vi "Autonomous Independent.vi"() -> ()   [LabVIEW 2014]
doc: "This VI is called when autonomous begins, and will automatically be terminated when autonomous ends. You can carry out timed or sensor driven robot movement independently without needing to return to the caller."
uses:
  <vilib>/addons/control/pid/pid.llb/PID Output Rate Limiter (DBL).vi
  <vilib>/addons/control/pid/NI_PID_pid.lvlib
panel:
  in  "Y 8":dbl
  in  "X 8":dbl format="%#_13g"
  in  "Forward_Drive_Time 2":dbl=2.55
  in  "Y 7":dbl=0.8
  in  "X 7":dbl format="%#_13g"
  in  "Max_Speed 2":dbl=1000.0 format="%#_13g"
  in  "Y 6":dbl
  in  "X 6":dbl format="%#_13g"
  in  "Container? y_t n_f":bool=TRUE
  in  "X 5":dbl format="%#_13g"
  in  "Y 5":dbl
  in  "Numeric":dbl=1781.0 format="%#_13g"
  in  "Max_Speed":dbl=1000.0 format="%#_13g"
  in  "Y 4":dbl
  in  "X 4":dbl format="%#_13g"
  in  "Forward_Drive_Time":dbl=2.8
  in  "Y 3":dbl=0.8
  in  "X 3":dbl format="%#_13g"
  in  "Stop":dbl=0.01
  in  "output rate (EGU/min)":dbl=25.0 format="%.2f"
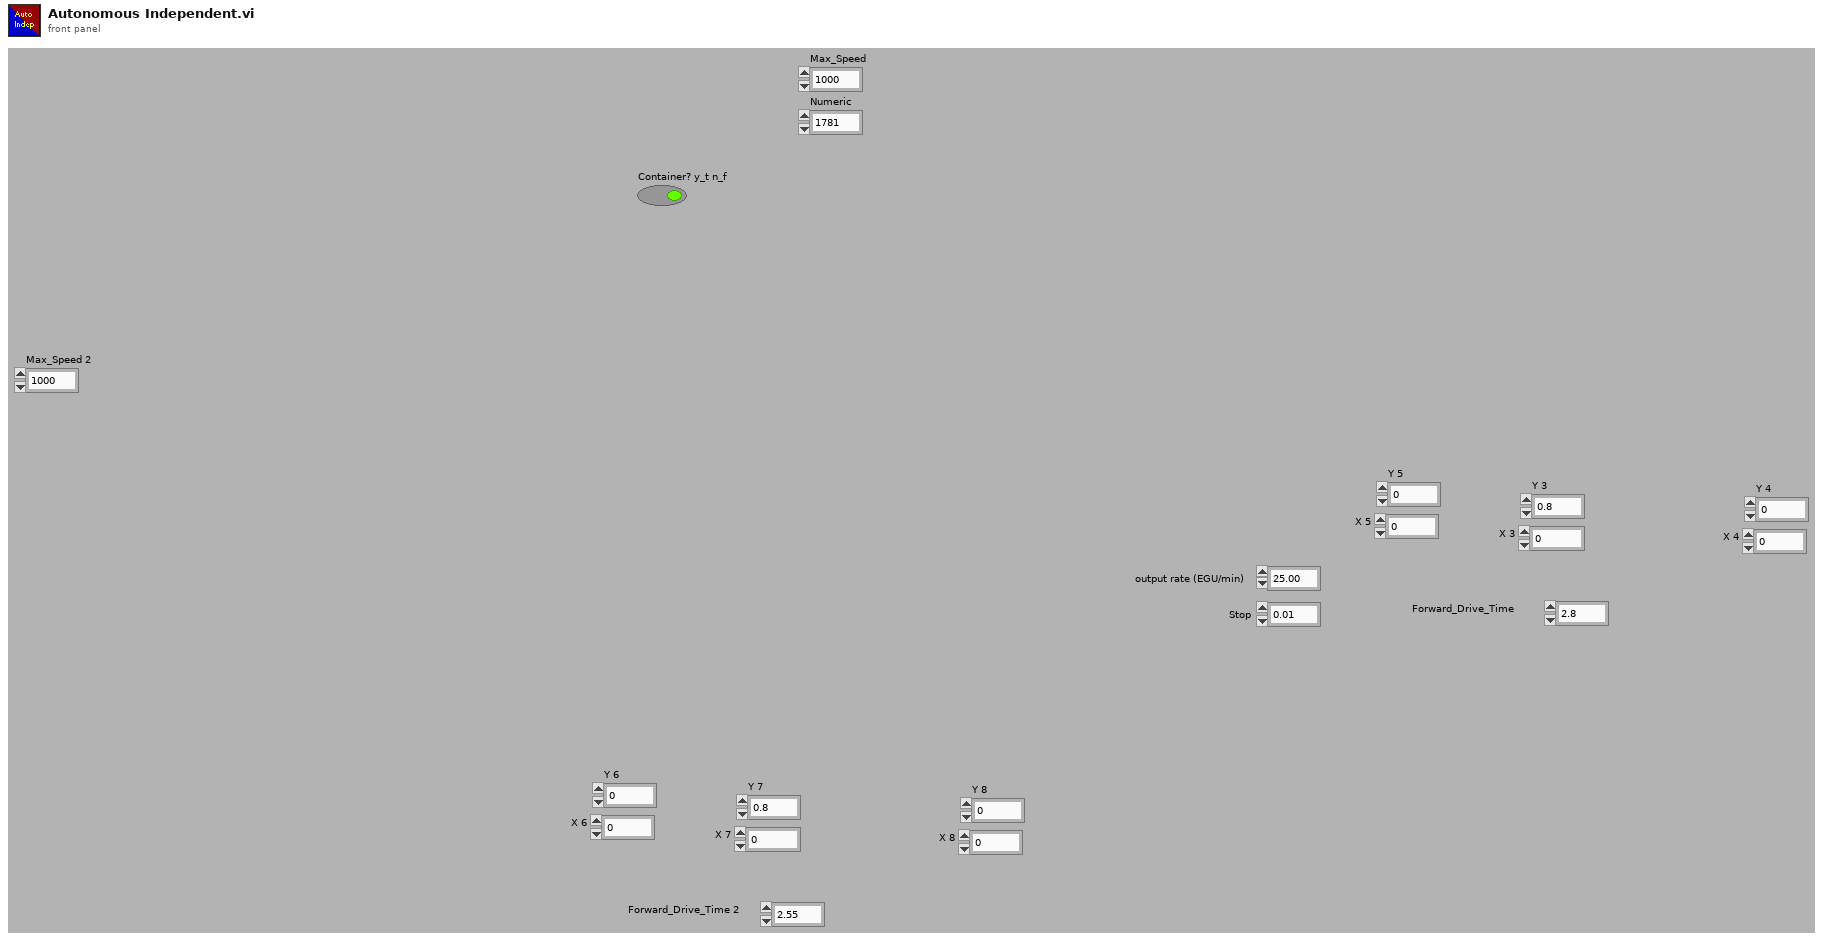
[diagram p1: front panel]
types:
  T1 = typedef "WPI_EncoderDevRef.ctl" = cluster{"DevStatus":errorcluster, "EncoderIndex":T2, "CounterIndex":T3, "DistancePerCount":dbl, "Decoding Type":T4}
  T2 = typedef "FPGA_EncoderIdx.ctl" = enum8{"Enc 0", "Enc 1", "Enc 2", "Enc 3", "Enc 4", "Enc 5", "Enc 6", "Enc 7", "Invalid"}
  T3 = typedef "FPGA_CounterCtrSystemIndex.ctl" = enum8{"Ctr 0", "Ctr 1", "Ctr 2", "Ctr 3", "Ctr 4", "Ctr 5", "Ctr 6", "Ctr 7", "Invalid"}
  T4 = typedef "WPI_EncoderType.ctl" = enum16{"1x", "2x", "4x"}
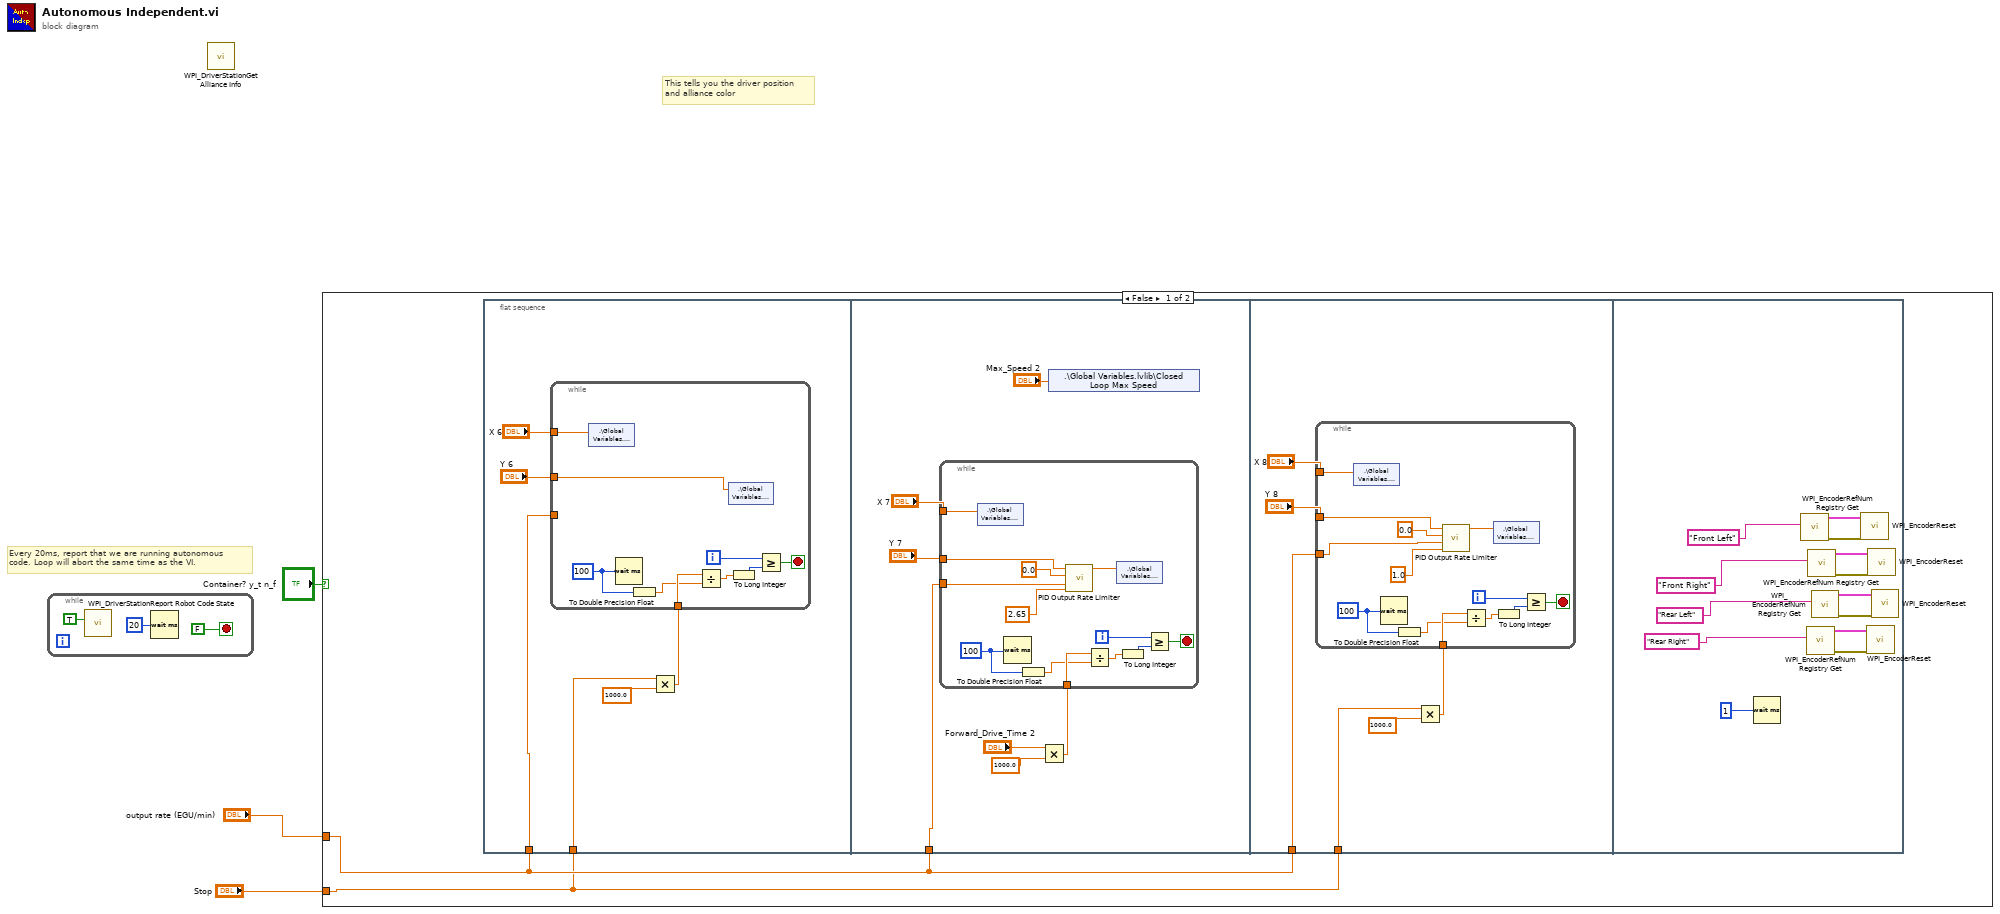
[diagram p0: block diagram]
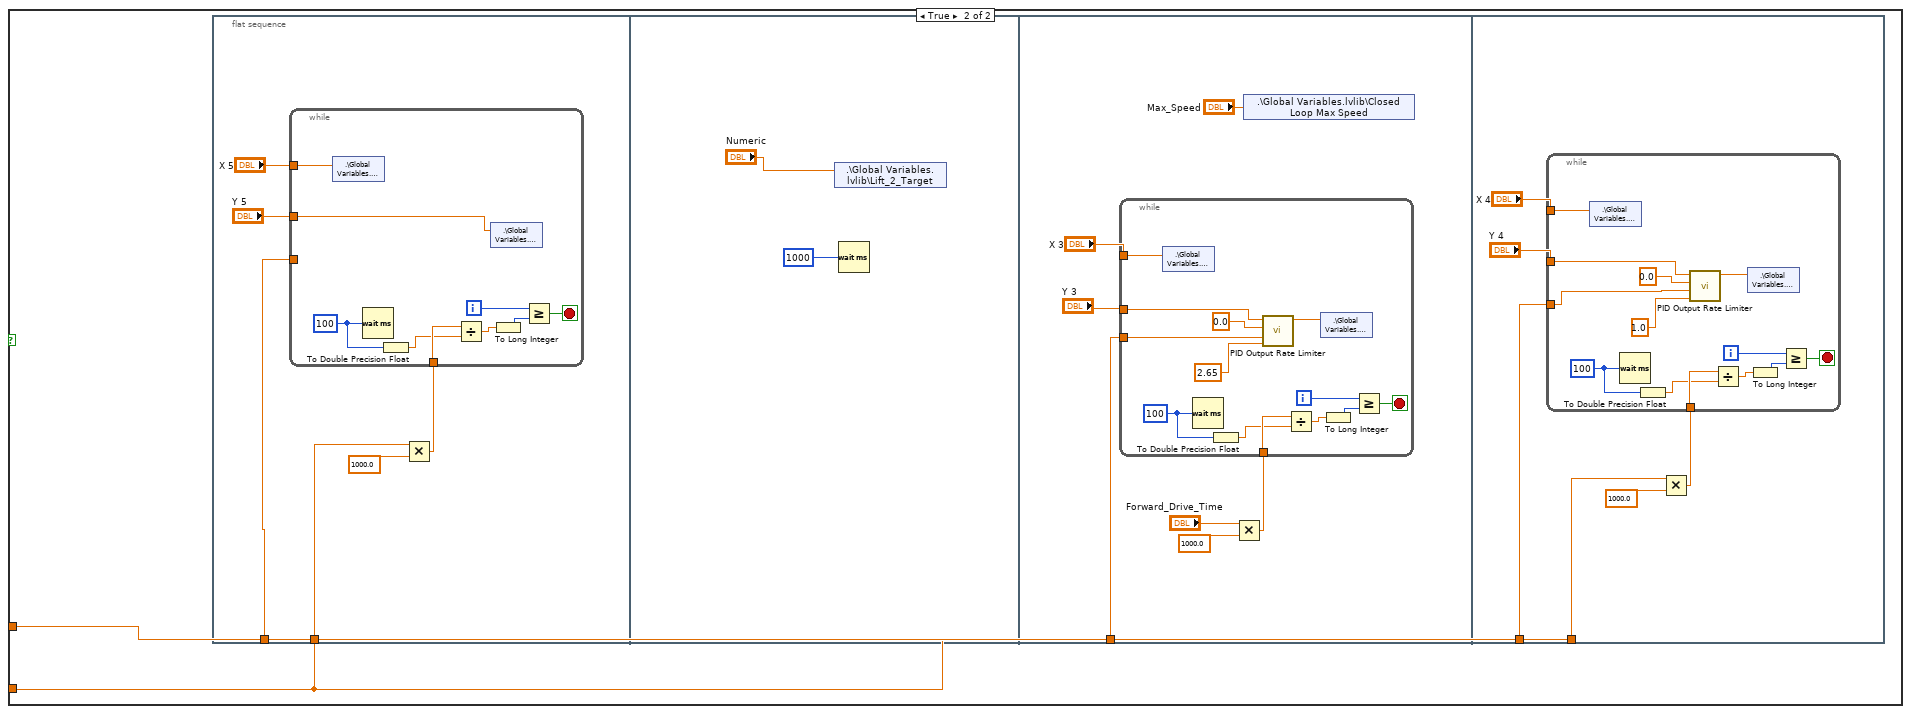
[diagram p2: hidden frame]
diagram:
  # "Every 20ms, report that we are running autonomous\ncode. Loop will abort the same time as the VI."
  # "This tells you the driver position\nand alliance color"
  n1 = while {
    stop <- FALSE stop-if-true
    n2 = call <vilib>:"WPI_DriverStationReport Robot Code State.vi"("Autonomous"=TRUE) -> ()  [unwired: 10 in, 1 out]
    n3 = Wait (ms)(milliseconds to wait=u32 20) -> ()  [unwired: 1 out]
  }
  n4 = call <vilib>:"WPI_DriverStationGet Alliance Info.vi"() -> ()  [unwired: 12 out]
  n5 = case shown="False" "Container? y_t n_f" {
    tunnel: "output rate (EGU/min)" -> [w8 w77]
    tunnel: "Stop" -> [w7 w76]
    frame False {
      n6 = flat-sequence {
        tunnel: w8 -> [w10]
        tunnel: w7 -> [w9]
        tunnel: w8 -> [w24]
        tunnel: w8 -> [w45]
        tunnel: w7 -> [w44]
        frame #0 {
          n7 = Multiply(x=w9, y=1000.0) -> (x*y=w13:dbl)
          n8 = while {
            tunnel: w13 -> [w21]
            tunnel: "X 6" -> [w16]
            tunnel: "Y 6" -> [w15]
            tunnel: w10 -> [_]
            i -> [w19]
            stop <- w23 stop-if-true
            w22 = u32 100 ("milliseconds to wait")
            n9 = shared-variable ".\\Global Variables.lvlib\\X"(w16) -> ()  [unwired: 1 in, 1 out]
            n10 = Wait (ms)(milliseconds to wait=w22) -> ()  [unwired: 1 out]
            n11 = To Double Precision Float(number=w22) -> (double precision float=w20:dbl)
            n12 = Divide(x=w21, y=w20) -> (x/y=w18:dbl)
            n13 = shared-variable ".\\Global Variables.lvlib\\Y"(w15) -> ()  [unwired: 1 in, 1 out]
            n14 = To Long Integer(number=w18) -> (32bit integer=w17:i32)
            n15 = Greater Or Equal?(x=w19, y=w17) -> (x >= y?=w23:bool)
          }
        }
        frame #1 {
          n16 = Multiply(x="Forward_Drive_Time 2", y=1000.0) -> (x*y=w27:dbl)
          n17 = while {
            tunnel: "Y 7" -> [w33]
            tunnel: w24 -> [w42]
            tunnel: w27 -> [w38]
            tunnel: "X 7" -> [w31]
            i -> [w36]
            stop <- w41 stop-if-true
            w39 = u32 100 ("milliseconds to wait")
            n18 = shared-variable ".\\Global Variables.lvlib\\X"(w31) -> ()  [unwired: 1 in, 1 out]
            n19 = Wait (ms)(milliseconds to wait=w39) -> ()  [unwired: 1 out]
            n20 = To Double Precision Float(number=w39) -> (double precision float=w37:dbl)
            n21 = call-poly <vilib>:"PID Output Rate Limiter.vi"("dt (s)"=2.65, "output rate (EGU/min)"=w42, "initial output"=0.0, "input (controller output)"=w33) -> ("output"=w32:dbl)  [unwired: 4 in, 1 out]
            n22 = Divide(x=w38, y=w37) -> (x/y=w35:dbl)
            n23 = shared-variable ".\\Global Variables.lvlib\\Y"(w32) -> ()  [unwired: 1 in, 1 out]
            n24 = To Long Integer(number=w35) -> (32bit integer=w34:i32)
            n25 = Greater Or Equal?(x=w36, y=w34) -> (x >= y?=w41:bool)
          }
          n26 = shared-variable ".\\Global Variables.lvlib\\Closed Loop Max Speed"("Max_Speed 2") -> ()  [unwired: 1 in, 1 out]
        }
        frame #2 {
          n27 = Multiply(x=w44, y=1000.0) -> (x*y=w48:dbl)
          n28 = while {
            tunnel: w48 -> [w58]
            tunnel: "X 8" -> [w52]
            tunnel: "Y 8" -> [w51]
            tunnel: w45 -> [w50]
            i -> [w56]
            stop <- w61 stop-if-true
            w59 = u32 100 ("milliseconds to wait")
            n29 = shared-variable ".\\Global Variables.lvlib\\X"(w52) -> ()  [unwired: 1 in, 1 out]
            n30 = Wait (ms)(milliseconds to wait=w59) -> ()  [unwired: 1 out]
            n31 = To Double Precision Float(number=w59) -> (double precision float=w57:dbl)
            n32 = call-poly <vilib>:"PID Output Rate Limiter.vi"("dt (s)"=1.0, "output rate (EGU/min)"=w50, "initial output"=0.0, "input (controller output)"=w51) -> ("output"=w53:dbl)  [unwired: 4 in, 1 out]
            n33 = Divide(x=w58, y=w57) -> (x/y=w55:dbl)
            n34 = shared-variable ".\\Global Variables.lvlib\\Y"(w53) -> ()  [unwired: 1 in, 1 out]
            n35 = To Long Integer(number=w55) -> (32bit integer=w54:i32)
            n36 = Greater Or Equal?(x=w56, y=w54) -> (x >= y?=w61:bool)
          }
        }
        frame #3 {
          n37 = Wait (ms)(milliseconds to wait=u32 1) -> ()  [unwired: 1 out]
          n38 = call <vilib>:"WPI_EncoderRefNum Registry Get.vi"("refnum name"="Front Left") -> ("error out"=w69:errorcluster, "EncoderDevRef"=w64:T1)  [unwired: 9 in]
          n39 = call <vilib>:"WPI_EncoderRefNum Registry Get.vi"("refnum name"="Rear Right") -> ("error out"=w71:errorcluster, "EncoderDevRef"=w70:T1)  [unwired: 9 in]
          n40 = call <vilib>:"WPI_EncoderRefNum Registry Get.vi"("refnum name"="Front Right") -> ("error out"=w73:errorcluster, "EncoderDevRef"=w72:T1)  [unwired: 9 in]
          n41 = call <vilib>:"WPI_EncoderRefNum Registry Get.vi"("refnum name"="Rear Left") -> ("error out"=w74:errorcluster, "EncoderDevRef"=w75:T1)  [unwired: 9 in]
          n42 = call <vilib>:"WPI_EncoderReset.vi"("error in (no error)"=w69, "EncoderDevRef"=w64) -> ()  [unwired: 8 in, 2 out]
          n43 = call <vilib>:"WPI_EncoderReset.vi"("error in (no error)"=w71, "EncoderDevRef"=w70) -> ()  [unwired: 8 in, 2 out]
          n44 = call <vilib>:"WPI_EncoderReset.vi"("error in (no error)"=w73, "EncoderDevRef"=w72) -> ()  [unwired: 8 in, 2 out]
          n45 = call <vilib>:"WPI_EncoderReset.vi"("error in (no error)"=w74, "EncoderDevRef"=w75) -> ()  [unwired: 8 in, 2 out]
        }
      }
    }
    frame True {
      n46 = flat-sequence {
        tunnel: w77 -> [w79]
        tunnel: w76 -> [w78]
        tunnel: w77 -> [w96]
        tunnel: w77 -> [w116]
        tunnel: w76 -> [w115]
        frame #0 {
          n47 = Multiply(x=w78, y=1000.0) -> (x*y=w82:dbl)
          n48 = while {
            tunnel: w82 -> [w90]
            tunnel: "X 5" -> [w85]
            tunnel: "Y 5" -> [w84]
            tunnel: w79 -> [_]
            i -> [w88]
            stop <- w92 stop-if-true
            w91 = u32 100 ("milliseconds to wait")
            n49 = shared-variable ".\\Global Variables.lvlib\\X"(w85) -> ()  [unwired: 1 in, 1 out]
            n50 = Wait (ms)(milliseconds to wait=w91) -> ()  [unwired: 1 out]
            n51 = To Double Precision Float(number=w91) -> (double precision float=w89:dbl)
            n52 = Divide(x=w90, y=w89) -> (x/y=w87:dbl)
            n53 = shared-variable ".\\Global Variables.lvlib\\Y"(w84) -> ()  [unwired: 1 in, 1 out]
            n54 = To Long Integer(number=w87) -> (32bit integer=w86:i32)
            n55 = Greater Or Equal?(x=w88, y=w86) -> (x >= y?=w92:bool)
          }
        }
        frame #1 {
          n56 = shared-variable ".\\Global Variables.lvlib\\Lift_2_Target"("Numeric") -> ()  [unwired: 1 in, 1 out]
          n57 = Wait (ms)(milliseconds to wait=u32 1000) -> ()  [unwired: 1 out]
        }
        frame #2 {
          n58 = Multiply(x="Forward_Drive_Time", y=1000.0) -> (x*y=w98:dbl)
          n59 = while {
            tunnel: "Y 3" -> [w104]
            tunnel: w96 -> [w113]
            tunnel: w98 -> [w109]
            tunnel: "X 3" -> [w102]
            i -> [w107]
            stop <- w112 stop-if-true
            w110 = u32 100 ("milliseconds to wait")
            n60 = shared-variable ".\\Global Variables.lvlib\\X"(w102) -> ()  [unwired: 1 in, 1 out]
            n61 = Wait (ms)(milliseconds to wait=w110) -> ()  [unwired: 1 out]
            n62 = To Double Precision Float(number=w110) -> (double precision float=w108:dbl)
            n63 = call-poly <vilib>:"PID Output Rate Limiter.vi"("dt (s)"=2.65, "output rate (EGU/min)"=w113, "initial output"=0.0, "input (controller output)"=w104) -> ("output"=w103:dbl)  [unwired: 4 in, 1 out]
            n64 = Divide(x=w109, y=w108) -> (x/y=w106:dbl)
            n65 = shared-variable ".\\Global Variables.lvlib\\Y"(w103) -> ()  [unwired: 1 in, 1 out]
            n66 = To Long Integer(number=w106) -> (32bit integer=w105:i32)
            n67 = Greater Or Equal?(x=w107, y=w105) -> (x >= y?=w112:bool)
          }
          n68 = shared-variable ".\\Global Variables.lvlib\\Closed Loop Max Speed"("Max_Speed") -> ()  [unwired: 1 in, 1 out]
        }
        frame #3 {
          n69 = Multiply(x=w115, y=1000.0) -> (x*y=w119:dbl)
          n70 = while {
            tunnel: w119 -> [w129]
            tunnel: "X 4" -> [w123]
            tunnel: "Y 4" -> [w122]
            tunnel: w116 -> [w121]
            i -> [w127]
            stop <- w132 stop-if-true
            w130 = u32 100 ("milliseconds to wait")
            n71 = shared-variable ".\\Global Variables.lvlib\\X"(w123) -> ()  [unwired: 1 in, 1 out]
            n72 = Wait (ms)(milliseconds to wait=w130) -> ()  [unwired: 1 out]
            n73 = To Double Precision Float(number=w130) -> (double precision float=w128:dbl)
            n74 = call-poly <vilib>:"PID Output Rate Limiter.vi"("dt (s)"=1.0, "output rate (EGU/min)"=w121, "initial output"=0.0, "input (controller output)"=w122) -> ("output"=w124:dbl)  [unwired: 4 in, 1 out]
            n75 = Divide(x=w129, y=w128) -> (x/y=w126:dbl)
            n76 = shared-variable ".\\Global Variables.lvlib\\Y"(w124) -> ()  [unwired: 1 in, 1 out]
            n77 = To Long Integer(number=w126) -> (32bit integer=w125:i32)
            n78 = Greater Or Equal?(x=w127, y=w125) -> (x >= y?=w132:bool)
          }
        }
      }
    }
  }
